vi "rotina_injecao_2.0.vi"() -> ()   [LabVIEW 2011]
panel:
  out "time string":string
  out "date string":string
  out "FID":cluster{"value":dbl}(graph)
  out "TCD":dbl(graph)
  in  "Counter":dbl=1.0
  in  "Stop":bool
  in  "Chromatogram Time (min)":dbl=1.0 caption="Time Target (s)"
  in  "Back Valve Time (min)":dbl=0.5 caption="Time Target (s)"
  out "?":bool
  out "Elapsed Time (min)":dbl caption="Elapsed Time (s)" format="%#_3g"
  in  "Cooling Down Time (min)":dbl=0.5000000000000001 caption="Time Target (s)"
  out "Start":bool
  in  "# Cicles":dbl=1.0
  out "Total Time (min)":dbl=1.0 caption="Time Target (s)"
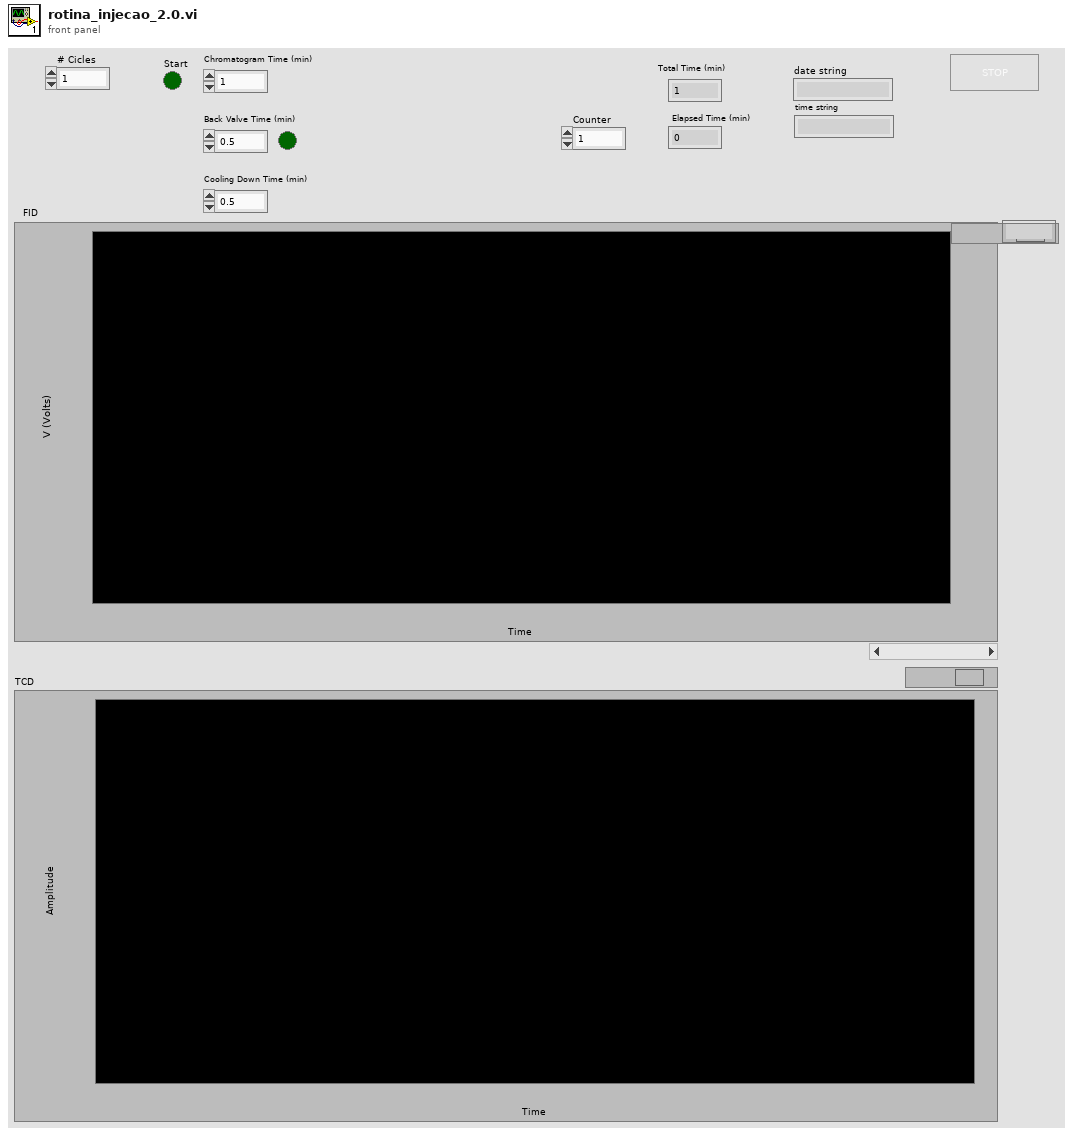
[diagram p1: front panel]
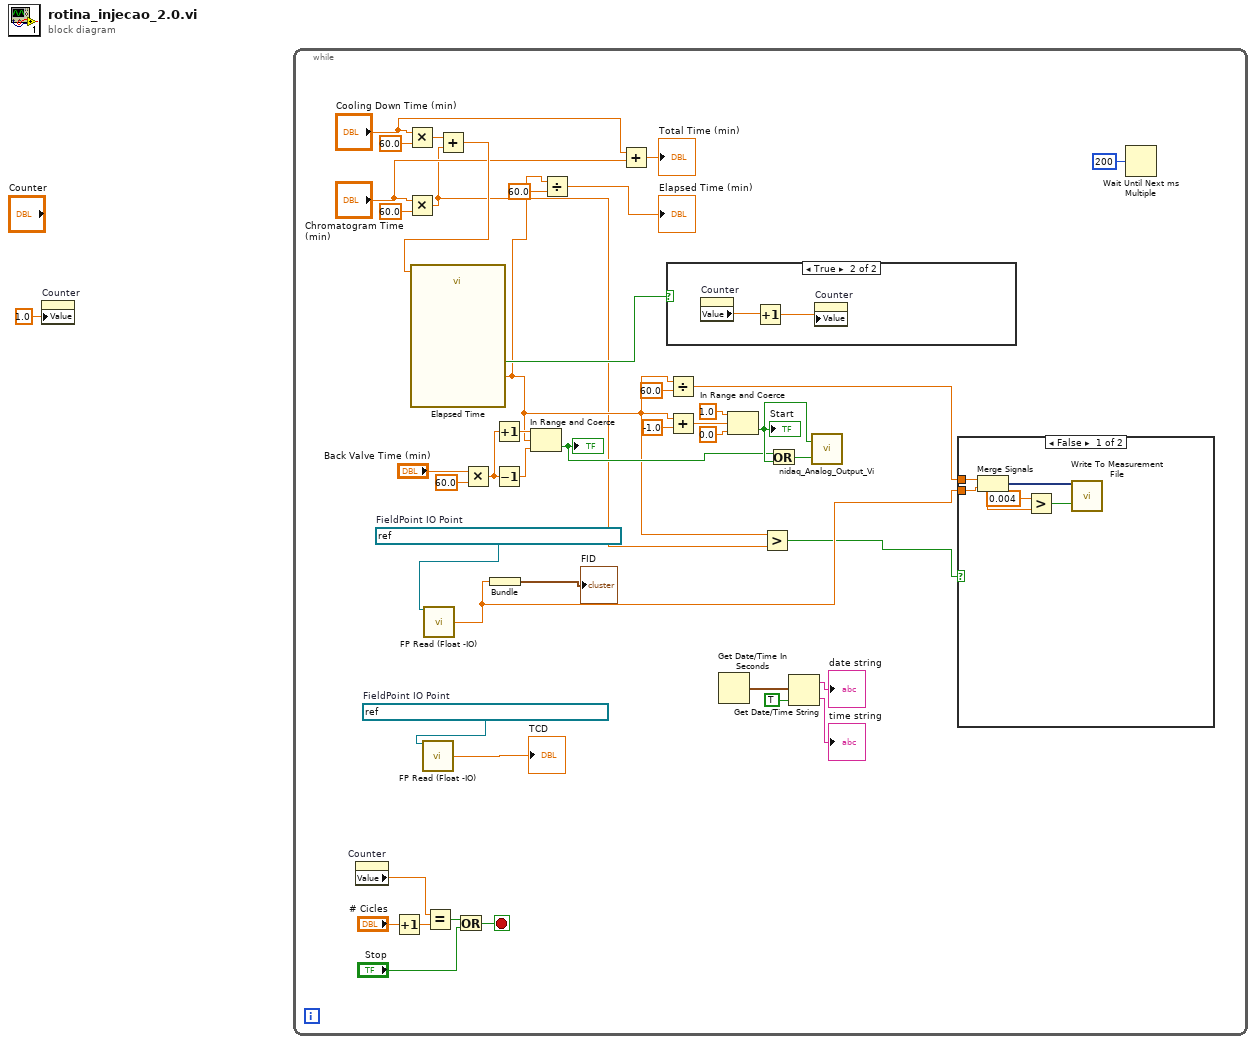
[diagram p0: block diagram]
diagram:
  n1 = property on="Counter" class="DigNum (strict)"("Value"=1.0 ("Counter")) -> ()  [unwired: 2 in, 2 out]
  n2 = while {
    stop <- w26 stop-if-true
    w24 = refnum<k21> "FieldPoint\\cfp2220\\cFP-AI-110 @4\\Channel 2"  # FieldPoint IO Point
    w25 = refnum<k21> "FieldPoint\\cfp2220\\cFP-AI-110 @4\\Channel 0"  # FieldPoint IO Point
    n3 = property on="Counter" class="DigNum (strict)"() -> ("Value"=w39:dbl)  [unwired: 2 in, 2 out]
    n4 = Increment(x="# Cicles") -> (x+1=w38:dbl)
    n5 = Multiply(x="Cooling Down Time (min)", y=60.0) -> (x*y=w40:dbl)
    n6 = Multiply(x="Chromatogram Time (min)", y=60.0) -> (x*y=w2:dbl)
    n7 = call <vilib>:"FP Read (Float -IO).vi"("FieldPoint IO Point In"=w24) -> ("value"=→"TCD":dbl)  [unwired: 11 in, 3 out]
    n8 = call <vilib>:"FP Read (Float -IO).vi"("FieldPoint IO Point In"=w25) -> ("value"=w17:dbl)  [unwired: 11 in, 3 out]
    n9 = Equal?(x=w39, y=w38) -> (x = y?=w36:bool)
    n10 = Add(x=w40, y=w2) -> (x+y=w31:dbl)
    n11 = call "Elapsed Time"("Time Target (s)"=w31) -> ("Elapsed Time (s)"=w3:dbl, "Time has Elapsed"=w16:bool)  [unwired: 11 in, 6 out]
    n12 = Or(x=w36, y="Stop") -> (x .or. y?=w26:bool)
    n13 = Multiply(x="Back Valve Time (min)", y=60.0) -> (x*y=w12:dbl)
    n14 = Bundle("value"=w17) -> (→"FID":cluster{"value":dbl})  [unwired: 1 out]
    n15 = Increment(x=w12) -> (x+1=w10:dbl)
    n16 = Decrement(x=w12) -> (x-1=w11:dbl)
    n17 = In Range and Coerce(upper limit=w10, x=w3, lower limit=w11) -> (In Range?=w13:bool)  [unwired: 1 out]
    "?" <- w13
    n18 = Divide(x=w3, y=60.0) -> (x/y=→"Elapsed Time (min)":dbl)
    n19 = Add(x="Cooling Down Time (min)", y="Chromatogram Time (min)") -> (x+y=→"Total Time (min)":dbl)
    n20 = case shown="True" w16 {
      frame False {
      }
      frame True {
        n21 = property on="Counter" class="DigNum (strict)"() -> ("Value"=w50:dbl)  [unwired: 2 in, 2 out]
        n22 = Increment(x=w50) -> (x+1=w51:dbl)
        n23 = property on="Counter" class="DigNum (strict)"("Value"=w51) -> ()  [unwired: 2 in, 2 out]
      }
    }
    n24 = Divide(x=w3, y=60.0) -> (x/y=w14:dbl)
    n25 = Add(x=w3, y=-1.0) -> (x+y=w34:dbl)
    n26 = Get Date/Time In Seconds() -> (seconds since 1Jan1904=w19:timestamp)
    n27 = In Range and Coerce(upper limit=1.0, x=w34, lower limit=0.0) -> (In Range?=w27:bool)  [unwired: 1 out]
    "Start" <- w27
    n28 = Greater?(x=w3, y=w2) -> (0:w5:bool)
    n29 = Or(x=w13, y=w27) -> (x .or. y?=w28:bool)
    n30 = Get Date/Time String(seconds (now)=w19, want seconds? (F)=TRUE) -> (date string=→"date string":string, time string=→"time string":string)  [unwired: 1 in]
    n31 = call "nidaq_Analog_Output_Vi.vi"("start Solenoide Valve"=w28, "start chromat"=w27) -> ()  [unwired: 1 in]
    n32 = case shown="False" w5 {
      tunnel: w14 -> [w46 _]
      tunnel: w17 -> [w48 _]
      frame False {
        n33 = Merge Signals(w46, w48) -> (w49:dynamicdata)
        n34 = Greater?(x=0.004, y=w46) -> (0:w45:bool)
        n35 = call "Write To Measurement File"("Signals"=w49, "new_file"=w45) -> ()  [unwired: 15 in, 3 out]
      }
      frame True {
      }
    }
    n36 = Wait Until Next ms Multiple(millisecond multiple=u32 200) -> ()  [unwired: 1 out]
  }
